vi "Initialize.vi"(8 "error in (no error)":errorcluster, 11 "VISA resource name":refnum<visa-resource-name>) -> (0 "error out":errorcluster, 2 "Instr ID":string, 3 "VISA resource name out":refnum<visa-resource-name>)   [LabVIEW 2023, in "Tti-Pl303Qmd.lvlib"]
doc: "Initialize Instrument - Get Instrument ID"
uses:
  Tti-Pl303Qmd.lvlib
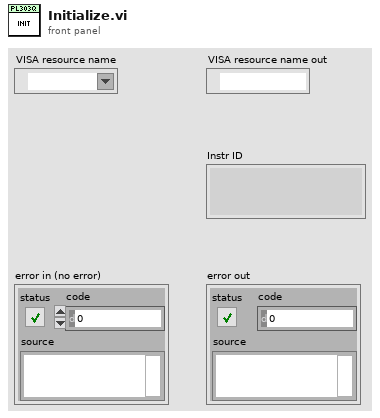
[diagram p1: front panel]
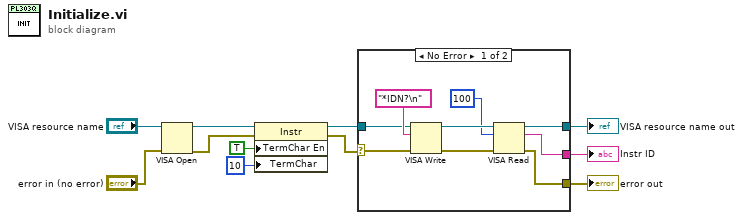
[diagram p0: block diagram]
diagram:
  n1 = VISA Open(error in (no error)="error in (no error)", VISA resource name="VISA resource name") -> (VISA resource name=w8:refnum<visa-resource-name>, error out=w4:errorcluster)  [unwired: 3 in]
  n2 = property class="Instr"(reference=w8, error in=w4, "TermChar En"=TRUE ("Message Based Settings:Termination Character Enable"), "TermChar"=u8 10 ("Message Based Settings:Termination Character")) -> (reference out=w5:refnum<visa-resource-name>, error out=w2:errorcluster)
  n3 = case shown="No Error" w2 {
    selector: w2 -> [w12 w22]
    tunnel: w5 -> [w13 w21]
    tunnel: [w16 w22] -> w11
    tunnel: [w18 w21] -> w7
    tunnel: [w15 _] -> w10
    frame No Error {
      n4 = VISA Write(VISA resource name=w13, write buffer="*IDN?\n", error in (no error)=w12) -> (VISA resource name out=w19:refnum<visa-resource-name>, error out=w17:errorcluster)  [unwired: 1 out]
      n5 = VISA Read(VISA resource name=w19, byte count=u32 100, error in (no error)=w17) -> (VISA resource name out=w18:refnum<visa-resource-name>, read buffer=w15:string, error out=w16:errorcluster)  [unwired: 1 out]
    }
    frame Error {
    }
  }
  "error out" <- w11
  "VISA resource name out" <- w7
  "Instr ID" <- w10
